vi "Coersion Dot.vi"() -> ()   [LabVIEW 2020]
panel:
  in  "u16 2":u16
  out "u8 2":u8
  out "u16":u16
  in  "u8":u8
  # "N"
  # "Rolled Off"
  # "255+N"
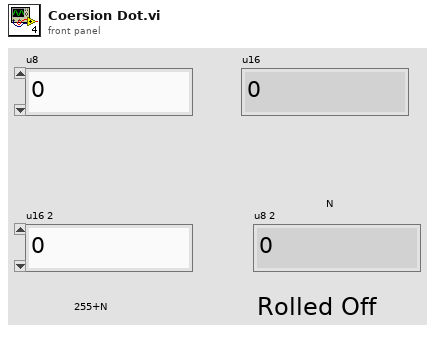
[diagram p1: front panel]
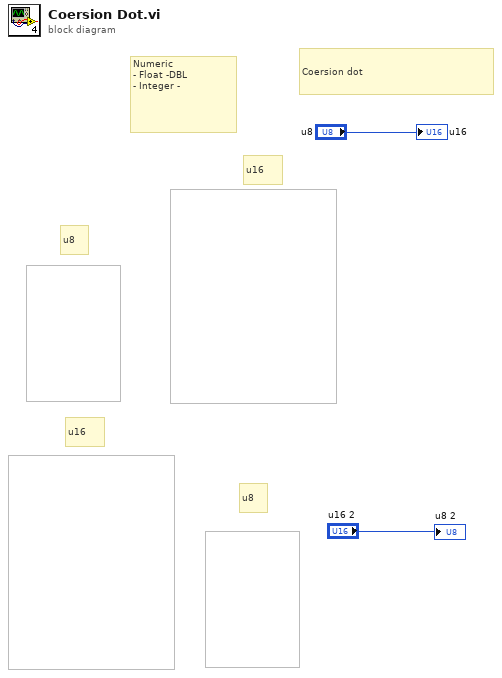
[diagram p0: block diagram]
diagram:
  # "Coersion dot"
  # "u8"
  # "u16"
  # "u16"
  # "u8"
  # "Numeric\n- Float -DBL\n- Integer -"
  "u16" <- "u8"
  "u8 2" <- "u16 2"
